vi "Do Check Available.vi"(8 "error in (no error)":errorcluster, 11 "output_actor_errorneous in":refnum<class "Output Actor Hardware.lvclass">) -> (0 "error out":errorcluster, 3 "output_actor_errorneous out":refnum<class "Output Actor Hardware.lvclass">)   [LabVIEW 2015, in "Output Actor Hardware.lvclass"]
uses:
  Output Actor Hardware.lvclass
  state.ctl
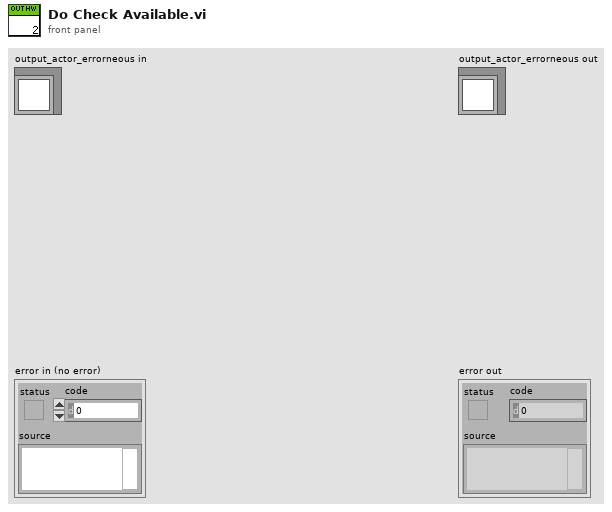
[diagram p1: front panel]
types:
  T1 = typedef "Output Actor Hardware.lvclass/state.ctl" = enum16{"not_available", "not_initialized", "ok"}
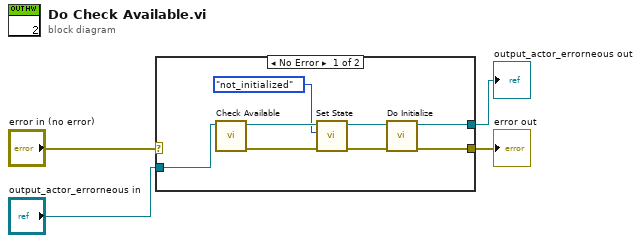
[diagram p0: block diagram]
diagram:
  n1 = case shown="No Error" "error in (no error)" {
    selector: "error in (no error)" -> [_ w14]
    tunnel: [w6 w14] -> w3
    tunnel: [w5 w13] -> w1
    tunnel: "output_actor_errorneous in" -> [w12 w13]
    frame No Error {
      n2 = call-dynamic "Check Available.vi"("Output Actor Hardware in"=w12) -> ("error out"=w11:errorcluster, "Output Actor Hardware out"=w10:refnum<class "Output Actor Hardware.lvclass">)  [unwired: 9 in]
      n3 = call "Set State.vi"("error in (no error)"=w11, "state"=state."not_initialized", "output_actor_errorneous in"=w10) -> ("error out"=w7:errorcluster, "output_actor_errorneous out"=w8:refnum<class "Output Actor Hardware.lvclass">)  [unwired: 7 in]
      n4 = call-dynamic "Do Initialize.vi"("error in (no error)"=w7, "output_actor_errorneous in"=w8) -> ("error out"=w6:errorcluster, "output_actor_errorneous out"=w5:refnum<class "Output Actor Hardware.lvclass">)  [unwired: 8 in]
    }
    frame Error {
    }
  }
  "error out" <- w3
  "output_actor_errorneous out" <- w1
